vi "set_debug.vi"(8 "error in (no error)":errorcluster, 11 "debug":bool) -> (0 "error out":errorcluster)   [LabVIEW 2024, in "Vision.lvlib"]
uses:
  Vision.lvlib
  bin/Vision.dll
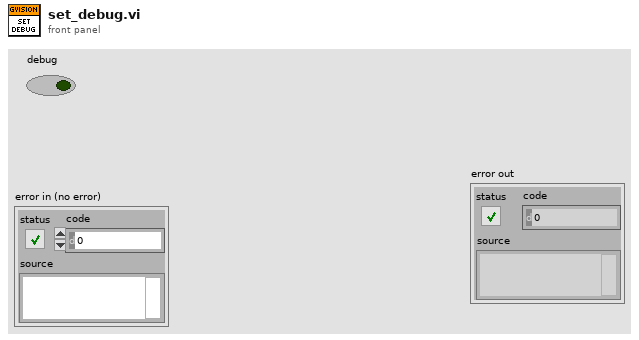
[diagram p1: front panel]
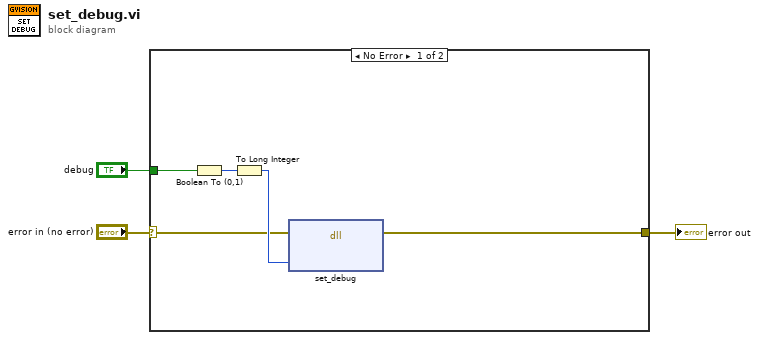
[diagram p0: block diagram]
diagram:
  n1 = case shown="No Error" "error in (no error)" {
    selector: "error in (no error)" -> [w5 w9]
    tunnel: [w4 w9] -> w2
    tunnel: "debug" -> [w8 _]
    frame No Error {
      n2 = Boolean To (0,1)(Boolean=w8) -> (0, 1=w7:i16)
      n3 = To Long Integer(number=w7) -> (32bit integer=w6:i32)
      n4 = dll-call lib="C:/Users/cfang/Desktop/nebraska-silicon-lab/pixel-gantry-control/Gantry/Shared Components/bin/Vision.dll" fn="set_debug"(error in=w5, "new_debug"=w6) -> (error out=w4:errorcluster)  [unwired: 4 in, 1 out]
    }
    frame Error {
    }
  }
  "error out" <- w2
